vi "Core.vi"(8 "error in (no error)":errorcluster, 10 "Actor in":refnum<class "Actor.lvclass">, 11 "Close File Msg in":refnum<class "Close File Msg.lvclass">) -> (0 "error out":errorcluster, 1 "Data":refnum<class "Data.lvclass">, 2 "Actor out":refnum<class "Actor.lvclass">, 3 "Close File Msg out":refnum<class "Close File Msg.lvclass">)   [LabVIEW 2020, in "File Writer.lvlib" / "Close File Msg.lvclass"]
doc: "Core of the Reponse Msg. Put the active code here.\n\nThe defaul implementation does nothing."
uses:
  Close File Msg.lvclass
  PPL/HDH.Data.Generic.lvlibp/Data.lvclass
  PPL/HDH.Actor Framework.Core.Actor.lvlibp/1abvi3w/vi.lib/ActorFramework/Actor/Actor.lvclass
  File Writer/File Writer.lvclass
  C:/Current projects/WS/PPL/HDH.Actor Framework.Core.Actor.lvlibp/1abvi3w/vi.lib/ActorFramework/Actor/Actor.lvclass
  Close File Msg.lvclass/Close File Msg.ctl
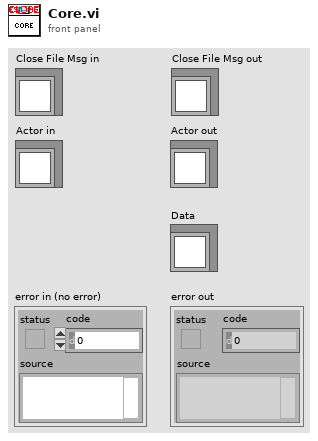
[diagram p1: front panel]
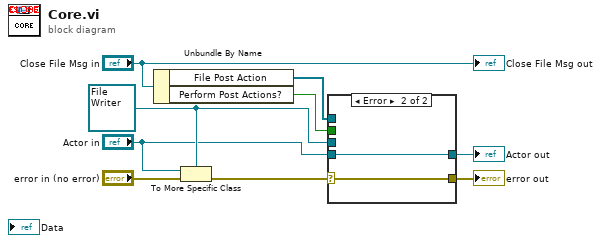
[diagram p0: block diagram]
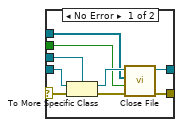
[diagram p2: hidden frame]
diagram:
  w8 = refnum<class "File Writer.lvclass"> refnum ("Actor in")
  n1 = Unbundle By Name("Close File Msg in") -> ("File Post Action"=w7:refnum<class "File Post Action.lvclass">[], "Perform Post Actions?"=w6:bool)
  n2 = To More Specific Class(target class=w8, reference="Actor in", error in="error in (no error)") -> (error out=w9:errorcluster)  [unwired: 1 out]
  n3 = case shown="Error" w9 {
    selector: w9 -> [w11 w20]
    tunnel: [w18 w20] -> w2
    tunnel: [w17 w19] -> w3
    tunnel: "Actor in" -> [w16 w19]
    tunnel: w8 -> [w15 _]
    tunnel: w7 -> [w13 _]
    tunnel: w6 -> [w12 _]
    frame No Error {
      n4 = To More Specific Class(target class=w15, reference=w16, error in=w11) -> (specific class reference=w14:refnum<class "File Writer.lvclass">, error out=w10:errorcluster)
      n5 = call "Close File.vi"("error in (no error)"=w10, "Perform Post Actions?"=w12, "File Post Action"=w13, "File Writer in"=w14) -> ("error out"=w18:errorcluster, "File Writer out"=w17:refnum<class "File Writer.lvclass">)  [unwired: 6 in]
    }
    frame Error {
    }
  }
  "error out" <- w2
  "Actor out" <- w3
  "Close File Msg out" <- "Close File Msg in"
